vi "Get Sections.vi"(11 "Dictionary in":refnum<class "Dictionary.lvclass">) -> (2 "OD Sections":refnum<class "Section.lvclass">[](array[class]), 3 "Dictionary out":refnum<class "Dictionary.lvclass">)   [LabVIEW 2024, in "Electronic Datasheet.lvlib" / "Dictionary.lvclass"]
uses:
  Dictionary.lvclass
  OD Section/Section.lvclass
  Dictionary.lvclass/Dictionary.ctl
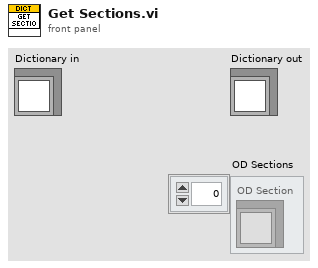
[diagram p1: front panel]
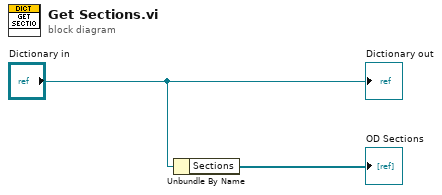
[diagram p0: block diagram]
diagram:
  n1 = Unbundle By Name("Dictionary in") -> ("Sections"=→"OD Sections":refnum<class "Section.lvclass">[])
  "Dictionary out" <- "Dictionary in"
